vi "Test Generate Mock Class Creates lvclass File.vi"(8 "error in (no error)":errorcluster, 11 "Test Case In":refnum<class "Pure Mock Class Generator Test.lvclass">) -> (0 "error out":errorcluster, 3 "Test Case Out":refnum<class "Pure Mock Class Generator Test.lvclass">)   [LabVIEW 2020, in "Pure Mock Class Generator Test.lvclass"]
uses:
  Pure Mock Class Generator Test.lvclass
  C:/Program Files (x86)/National Instruments/LabVIEW 2020/vi.lib/Astemes/LUnit/Test Case.lvclass
  <vilib>/Astemes/LUnit/Test Case.lvclass/Test Case.ctl
  <vilib>/Astemes/LUnit/Append Pass Result.vi
  <vilib>/Astemes/LUnit/Append Fail Result.vi
  <vilib>/Astemes/LUnit/Test Case.lvclass
  source/Scripting/Pure Mock Class Generator/Pure Mock Class Generator.lvclass
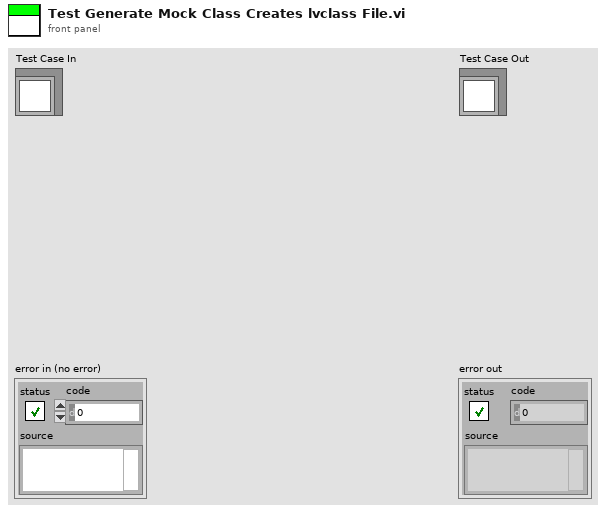
[diagram p1: front panel]
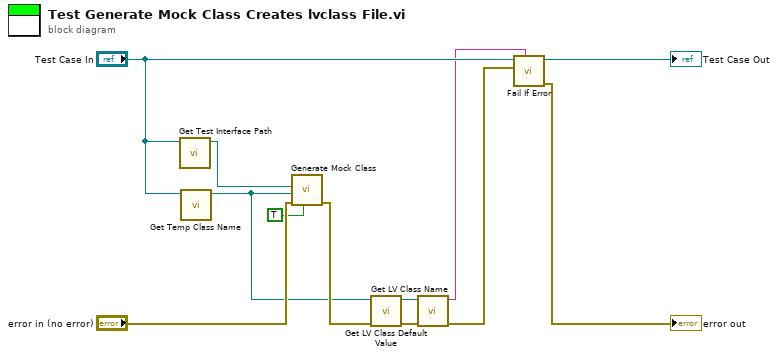
[diagram p0: block diagram]
diagram:
  n1 = call "Get Test Interface Path.vi"("Mock Class Generator Test in"="Test Case In") -> ("Test Class Path"=w10:path)  [unwired: 10 in]
  n2 = call "Get Temp Class Name.vi"("Mock Class Generator Test in"="Test Case In") -> ("Test Class Path"=w5:path)  [unwired: 10 in]
  n3 = call "Generate Mock Class.vi"("Add to lvproj?"=TRUE, "error in (no error)"="error in (no error)", "Destination Class Path"=w5, "Source Class Path"=w10) -> ("error out"=w7:errorcluster)  [unwired: 7 in]
  n4 = call <vilib>:"Get LV Class Default Value.vi"("error in (no error)"=w7, "class path"=w5) -> ("error out"=w6:errorcluster, "object"=w4:refnum<class>)  [unwired: 8 in]
  n5 = call <vilib>:"Get LV Class Name.vi"("error in (no error)"=w6, "object"=w4) -> ("error out"=w2:errorcluster, "class name"=w3:string)  [unwired: 8 in]
  n6 = call <vilib>:"Fail If Error.vi"("Description"=w3, "Assert error"=w2, "LUnit Test Case In"="Test Case In") -> ("error out"=→"error out":errorcluster, "LUnit Test Case Out"=→"Test Case Out":refnum<class "Pure Mock Class Generator Test.lvclass">)  [unwired: 7 in]
